vi "Main.vi"() -> ()   [LabVIEW 2013]
uses:
  Charge Settings TypeDef.ctl
panel:
  in  "Tab Control":T1(tab)
  in  "Stop C-D":bool
  in  "Start C-D":bool
  in  "Зарядка-разрядка":T2
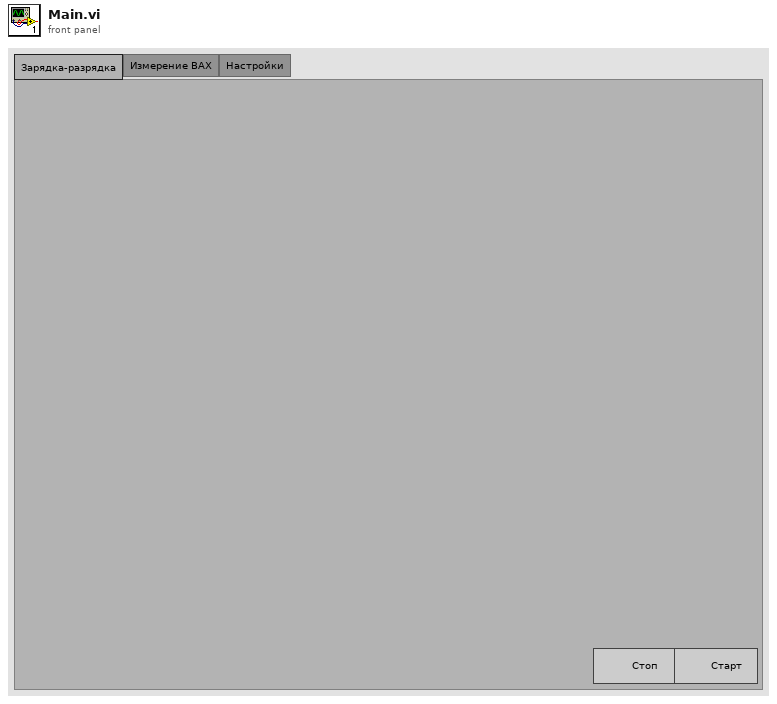
[diagram p1: front panel]
types:
  T1 = enum32{"Зарядка-разрядка", "Измерение ВАХ", "Настройки"}
  T2 = typedef "Charge Settings TypeDef.ctl" = cluster{"Current Input":tag, "Capacitor Voltage Input":tag, "Voltage Output":tag}
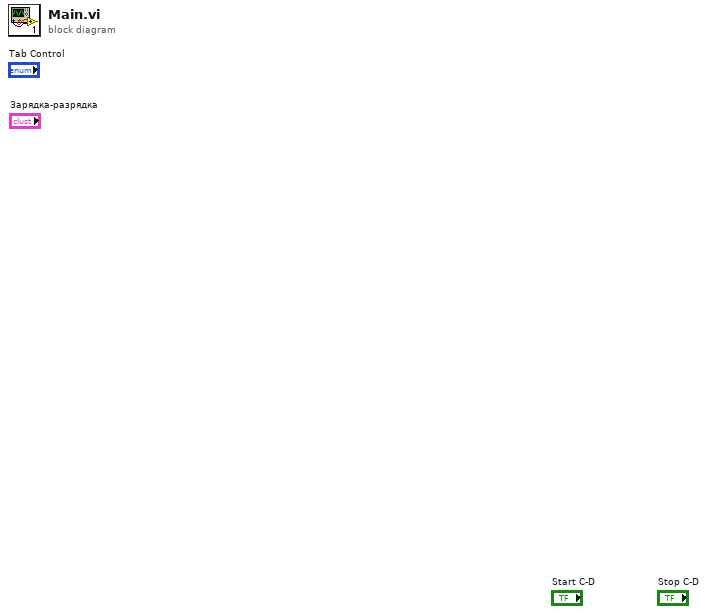
[diagram p0: block diagram]
diagram:
